vi "Init.vi"(7 "Target Enqueuer":refnum<class "Message Enqueuer.lvclass">, 8 "error in":errorcluster, 11 "HAL GOOP4:Series Base in":refnum<class "Series Base.lvclass">) -> (0 "error out":errorcluster, 3 "HAL GOOP4:Series Base out":refnum<class "Series Base.lvclass">)   [LabVIEW 2023, in "Series Base.lvclass"]
uses:
  Series Base.lvclass
  <vilib>/ActorFramework/Message Enqueuer/Message Enqueuer.lvclass
  Measure and Stimulus Subsystems/Measure and Stimulus Subsystems.lvclass
  Series Base.lvclass/Series Base.ctl
  4ad7cdfb-9af4-463b-909e-db929ec96591.vi
  <vilib>/JDP Science/JSONtext/Find Item.vi
  <vilib>/JDP Science/JSONtext/Next JSON Value.vi
  <vilib>/JDP Science/JSONtext/String Subset.vi
  <vilib>/JDP Science/JSONtext/Parsing/Advance past next JSON Value (inlined COPY).vi
  <vilib>/JDP Science/JSONtext/Parsing/Advance past whitespace.vi
  <vilib>/JDP Science/JSONtext/Parsing/Advance past String.vi
  <vilib>/JDP Science/JSONtext/Parsing/Advance past Number.vi
  <vilib>/JDP Science/JSONtext/Parsing/Advance past Line Ending.vi
  <vilib>/JDP Science/JSONtext/Parsing/Parse Full Path or Item Name.vi
  <vilib>/JDP Science/JSONtext/Parsing/Advance past Array.vi
  <vilib>/JDP Science/JSONtext/Parsing/Advance past Object.vi
  <vilib>/JDP Science/JSONtext/support/Error Cluster From Code.vi
  <vilib>/JDP Science/JSONtext/Offset/Find Item Locations by Path.vi
  <vilib>/JDP Science/JSONtext/JSON text to Variant.vi
  <vilib>/Utility/error.llb/Error Cluster From Error Code.vi
  <vilib>/JDP Science/JSONtext/LVClass Serializer/JSONtext LVClass Serializer.lvclass
  <vilib>/ErrorRing/Error Ring.xnode
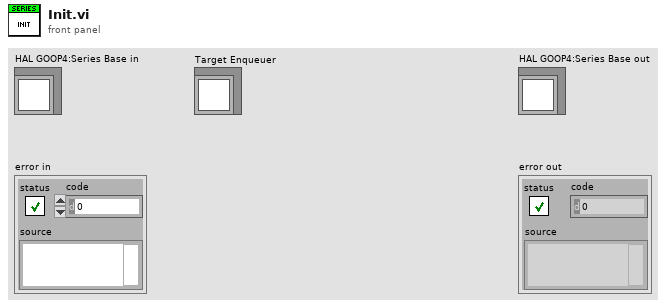
[diagram p1: front panel]
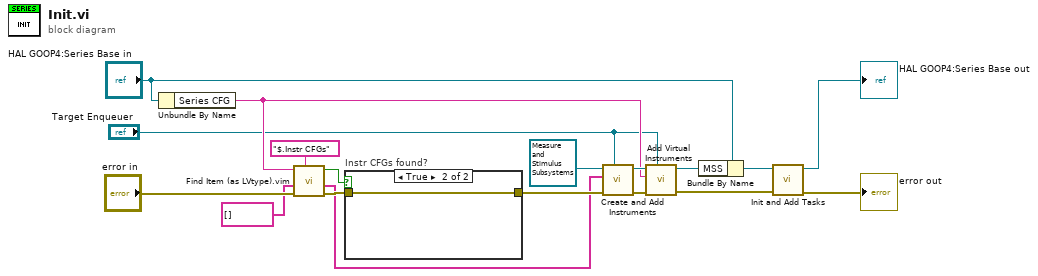
[diagram p0: block diagram]
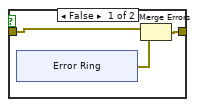
[diagram p2: hidden frame]
diagram:
  n1 = Unbundle By Name("HAL GOOP4:Series Base in") -> ("Series CFG"=w3:string)
  n2 = call "Find Item (as LVtype).vim"("$Path or Item Name"="$.Instr CFGs", "error in (no error)"="error in", "Data Type and Default Value"=string[] [], "JSON"=w3) -> ("error out"=w6:errorcluster, "Data"=w2:string[], "Found"=w7:bool)  [unwired: 4 in, 1 out]
  n3 = case "Instr CFGs found?" shown="True" w7 {
    tunnel: w6 -> [w20 w27]
    tunnel: [w21 w27] -> w5
    frame False {
      n4 = xnode "Error Ring"() -> ("error out"=w19:errorcluster)
      n5 = Merge Errors(w20, w19) -> (w21:errorcluster)
    }
    frame True {
    }
  }
  n6 = call "Create and Add Instruments.vi"("Target Enqueuer"="Target Enqueuer", "Error In"=w5, "Physical Intr CFGs"=w2, "MSS in"=refnum<class "Measure and Stimulus Subsystems.lvclass"> refnum ("Host MSS")) -> ("Error Out"=w18:errorcluster, "MSS out"=w17:refnum<class "Measure and Stimulus Subsystems.lvclass">)  [unwired: 6 in]
  n7 = call "Add Virtual Instruments.vi"("Enqueuer"="Target Enqueuer", "error in"=w18, "<JSON CFG>"=w3, "MSS in"=w17) -> ("error out"=w16:errorcluster, "MSS out"=w13:refnum<class "Measure and Stimulus Subsystems.lvclass">)  [unwired: 6 in]
  n8 = Bundle By Name(cluster="HAL GOOP4:Series Base in", "MSS"=w13) -> (w12:refnum<class "Series Base.lvclass">)
  n9 = call-dynamic "Init and Add Tasks.vi"("error in (no error)"=w16, "HAL GOOP4:Series Base in"=w12) -> ("error out"=→"error out":errorcluster, "HAL GOOP4:Series Base out"=→"HAL GOOP4:Series Base out":refnum<class "Series Base.lvclass">)  [unwired: 8 in]
